vi "OldClimbExecute.vi"(8 "error in (no error)":errorcluster) -> (0 "error out":errorcluster)   [LabVIEW 2023]
uses:
  <vilib>/Rock Robotics/WPI/ThirdParty/JAS_Junk/TrajLib/Trajectory_Library.lvlib
  OldClimbNetworkingGlobal.vi
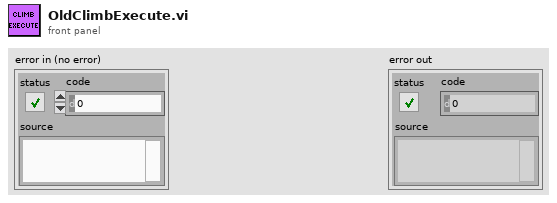
[diagram p1: front panel]
types:
  T1 = typedef "WPI_MotorControlDeviceRef.ctl" = cluster{"DeviceStatus":errorcluster, "Type":T2, "PWM":cluster{"PWM Channel":T3, "DeadBand":T4}, "CAN":cluster{"Device Number":u8, "SetOutput VI Ref":variant, "GetOutput VI Ref":variant, "Enable VI Ref":variant, "Disable VI Ref":variant, "Data":variant}, "Invert":bool, "DIO PWM":cluster{"PWM \"Enable\" Channel":T3, "DIOChannel":T5, "PWM Rate":dbl}}
  T2 = typedef "WPI_MotorControlType.ctl" = enum16{"PWM", "CAN", "DIO PWM"}
  T3 = typedef "FPGA_DIOPWMChannel.ctl" = enum8{"PWM 0", "PWM 1", "PWM 2", "PWM 3", "PWM 4", "PWM 5", "PWM 6", "PWM 7", "PWM 8", "PWM 9", "PWM MXP 0", "PWM MXP 1", "PWM MXP 2", "PWM MXP 3", "PWM MXP 4", "PWM MXP 5", "PWM MXP 6", "PWM MXP 7", "PWM MXP 8", "PWM MXP 9", "Invalid"}
  T4 = typedef "WPI_PWMDeadband.ctl" = cluster{"Name":string, "maxPositivePwm":i32, "minPositivePwm":i32, "centerPwm":i32, "maxNegativePwm":i32, "minNegativePwm":i32, "angularRange":u16}
  T5 = typedef "FPGA_DIOChannel.ctl" = enum8{"DIO 0", "DIO 1", "DIO 2", "DIO 3", "DIO 4", "DIO 5", "DIO 6", "DIO 7", "DIO 8", "DIO 9", "DIO MXP 0", "DIO MXP 1", "DIO MXP 2", "DIO MXP 3", "DIO MXP 4", "DIO MXP 5", "DIO MXP 6", "DIO MXP 7", "DIO MXP 8", "DIO MXP 9", "DIO MXP 10", "DIO MXP 11", "DIO MXP 12", "DIO MXP 13", "DIO MXP 14", "DIO MXP 15", "SPI Port CS1", "SPI Port CS2", "SPI Port CS3", "SPI Port MISO", "SPI Port MOSI", "Invalid"}
  T6 = typedef "Trajectory_Library.lvlib/PosCtrl_Tuning_Type.ctl" = cluster{"Slope":dbl, "Offset":dbl, "Error Deadband":dbl, "At Reference Count":i32, "Negate Output":bool, "Max Allowd Position":dbl, "Min Allowd Position":dbl}
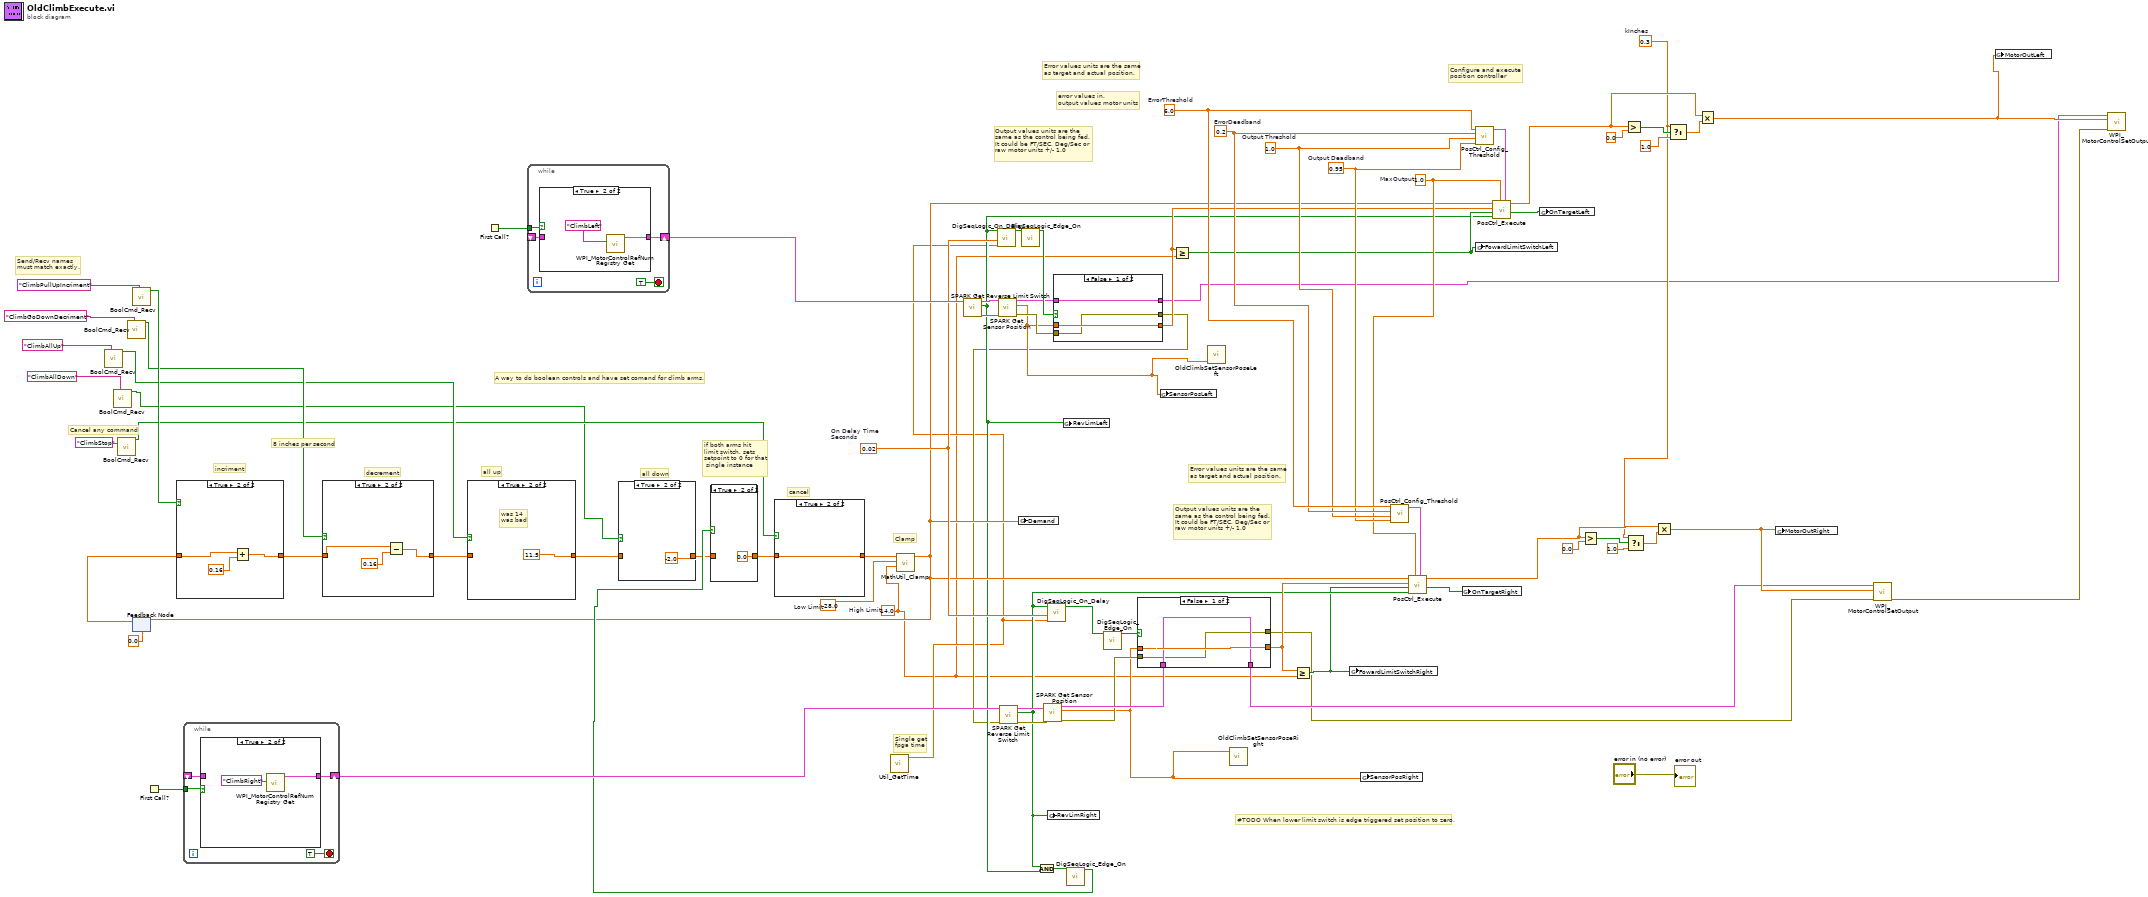
[diagram p0: block diagram]
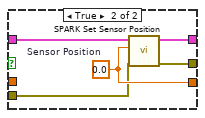
[diagram p5: hidden frame]
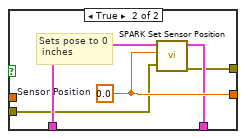
[diagram p6: hidden frame]
diagram:
  w1 = 14.0  # High Limit
  w30 = 0.3  # kInches
  w46 = 0.02  # On Delay Time Seconds
  w62 = -28.0  # Low Limit
  w49 = 1.0  # MaxOutput
  w53 = 6.0  # ErrorThreshold
  w52 = 0.2  # ErrorDeadband
  w51 = 1.0  # Output Threshold
  w50 = 0.95  # Output Deadband
  # "Single get\nfpga time"
  # "if both arms hit \nlimit switch, sets \nsetpoint to 0 for that\n single instance"
  # "#TODO When lower limit switch is edge triggered set position to zero."
  # "cancel"
  # "Clamp"
  # "8 inches per second"
  # "all down"
  # "all up"
  # "decrement"
  # "incriment"
  # "Cancel any command"
  # "Send/Recv names\nmust match exactly."
  # "A way to do boolean controls and have set comand for climb arms."
  # "error values in.\noutput values motor units"
  # "Output values units are the\nsame as the control being fed.  \nIt could be FT/SEC, Deg/Sec or\nraw motor units +/- 1.0"
  # "Error values units are the same \nas target and actual position."
  # "Output values units are the\nsame as the control being fed.  \nIt could be FT/SEC, Deg/Sec or\nraw motor units +/- 1.0"
  # "Error values units are the same \nas target and actual position."
  # "Configure and execute \nposition controller"
  n1 = call <vilib>:"BoolCmd_Recv.vi"("Command Name"="ClimbAllUp") -> ("New Request"=w58:bool)  [unwired: 9 in, 1 out]
  n2 = call <vilib>:"BoolCmd_Recv.vi"("Command Name"="ClimbAllDown") -> ("New Request"=w27:bool)  [unwired: 9 in, 1 out]
  n3 = call <vilib>:"BoolCmd_Recv.vi"("Command Name"="ClimbStop") -> ("New Request"=w57:bool)  [unwired: 9 in, 1 out]
  n4 = call <vilib>:"BoolCmd_Recv.vi"("Command Name"="ClimbGoDownDecriment") -> ("New Request"=w59:bool)  [unwired: 9 in, 1 out]
  n5 = call <vilib>:"BoolCmd_Recv.vi"("Command Name"="ClimbPullUpIncriment") -> ("New Request"=w60:bool)  [unwired: 9 in, 1 out]
  n6 = feedback #1(0.0 ("false")) -> (w66:dbl)
  n7 = First Call?() -> (First Call?: T/F=w24:bool)
  n8 = case shown="True" w60 {
    tunnel: w66 -> [w78 w81]
    tunnel: [w78 w79] -> w65
    frame False {
    }
    frame True {
      n9 = Add(x=w81, y=0.16) -> (x+y=w79:dbl)
    }
  }
  n10 = while {
    tunnel: w24 -> [w84]
    shift-right: [w85] -> w75
    shift-left: _ -> [w83]
    stop <- TRUE stop-if-true
    n11 = case shown="True" w84 {
      tunnel: [w86 w88] -> w85
      tunnel: w83 -> [w86 _]
      frame False {
      }
      frame True {
        n12 = call <vilib>:"WPI_MotorControlRefNum Registry Get.vi"("refnum name"="ClimbRight") -> ("MotorControlDevRef"=w88:T1)  [unwired: 9 in, 1 out]
      }
    }
  }
  n13 = case shown="True" w59 {
    tunnel: w65 -> [w89 w91]
    tunnel: [w89 w90] -> w64
    frame False {
    }
    frame True {
      n14 = Subtract(x=w91, y=0.16) -> (x-y=w90:dbl)
    }
  }
  n15 = case shown="True" w58 {
    tunnel: w64 -> [w93 _]
    tunnel: [w93 11.5 ("y")] -> w63
    frame False {
    }
    frame True {
      # "was 14\nwas bad"
    }
  }
  n16 = First Call?() -> (First Call?: T/F=w23:bool)
  n17 = while {
    tunnel: w23 -> [w97]
    shift-right: [w98] -> w76
    shift-left: _ -> [w96]
    stop <- TRUE stop-if-true
    n18 = case shown="True" w97 {
      tunnel: [w99 w101] -> w98
      tunnel: w96 -> [w99 _]
      frame False {
      }
      frame True {
        n19 = call <vilib>:"WPI_MotorControlRefNum Registry Get.vi"("refnum name"="ClimbLeft") -> ("MotorControlDevRef"=w101:T1)  [unwired: 9 in, 1 out]
      }
    }
  }
  n20 = case shown="True" w27 {
    tunnel: w63 -> [w102 _]
    tunnel: [w102 -2.0 ("y")] -> w26
    frame False {
    }
    frame True {
    }
  }
  n21 = call <vilib>:"Util_GetTime.vi"() -> ("FPGA_Time_Seconds"=w2:dbl)  [unwired: 9 in, 2 out]
  n22 = call <vilib>:"SPARK Get Reverse Limit Switch.vi"("MotorControlDevRef in"=w76) -> ("error out"=w21:errorcluster, "Hard Limit Rev"=w8:bool, "MotorControlDevRef out"=w43:T1)  [unwired: 7 in, 1 out]
  n23 = call <vilib>:"DigSeqLogic_On_Delay.vi"("Time"=w2, "Delay"=w46, "Input"=w8) -> ("Output"=w45:bool)  [unwired: 7 in, 1 out]
  n24 = call <vilib>:"SPARK Get Sensor Position.vi"("error in (no error)"=w21, "MotorControlDevRef in"=w43) -> ("error out"=w20:errorcluster, "Sensor Position"=w7:dbl, "MotorControlDevRef out"=w42:T1)  [unwired: 6 in, 1 out]
  n25 = call <vilib>:"DigSeqLogic_Edge_On.vi"("Input"=w45) -> ("On Edge"=w44:bool)  [unwired: 10 in]
  n26 = case shown="False" w44 {
    tunnel: w42 -> [w106 w111]
    tunnel: [w106 w110] -> w4
    tunnel: w7 -> [w105 _]
    tunnel: [w105 w109] -> w41
    tunnel: w20 -> [w104 w108]
    tunnel: [w104 w107] -> w3
    frame False {
    }
    frame True {
      w109 = 0.0  # Sensor Position
      n27 = call <vilib>:"SPARK Set Sensor Position.vi"("error in"=w108, "Position"=w109, "MotorControlDeviceRef"=w111) -> ("error out"=w107:errorcluster, "MotorControlDeviceRef"=w110:T1)  [unwired: 7 in]
    }
  }
  n28 = call <vilib>:"SPARK Get Reverse Limit Switch.vi"("error in (no error)"=w3, "MotorControlDevRef in"=w75) -> ("error out"=w19:errorcluster, "Hard Limit Rev"=w17:bool, "MotorControlDevRef out"=w74:T1)  [unwired: 6 in, 1 out]
  n29 = And(x=w17, y=w8) -> (x .and. y?=w29:bool)
  n30 = call <vilib>:"SPARK Get Sensor Position.vi"("error in (no error)"=w19, "MotorControlDevRef in"=w74) -> ("error out"=w18:errorcluster, "Sensor Position"=w16:dbl, "MotorControlDevRef out"=w47:T1)  [unwired: 6 in, 1 out]
  n31 = call <vilib>:"DigSeqLogic_On_Delay.vi"("Time"=w2, "Delay"=w46, "Input"=w17) -> ("Output"=w55:bool)  [unwired: 7 in, 1 out]
  n32 = global write "OldClimbNetworkingGlobal.vi" "RevLimRight"(w17) -> ()
  n33 = global write "OldClimbNetworkingGlobal.vi" "RevLimLeft"(w8) -> ()
  n34 = call <vilib>:"DigSeqLogic_Edge_On.vi"("Input"=w29) -> ("On Edge"=w28:bool)  [unwired: 10 in]
  n35 = case shown="True" w28 {
    tunnel: w26 -> [w112 _]
    tunnel: [w112 0.0 ("y")] -> w25
    frame False {
    }
    frame True {
    }
  }
  n36 = case shown="True" w57 {
    tunnel: w25 -> [w114 w115]
    tunnel: [w114 w115] -> w61
    frame False {
    }
    frame True {
    }
  }
  n37 = call <vilib>:"MathUtil_Clamp.vi"("High Limit"=w1, "Low Limit"=w62, "Value"=w61) -> ("Result"=w9:dbl)  [unwired: 8 in]
  n38 = feedback-in #1(w9) -> ()
  n39 = global write "OldClimbNetworkingGlobal.vi" "Demand"(w9) -> ()
  n40 = call <vilib>:"DigSeqLogic_Edge_On.vi"("Input"=w55) -> ("On Edge"=w48:bool)  [unwired: 10 in]
  n41 = case shown="False" w48 {
    tunnel: w16 -> [w118 _]
    tunnel: [w118 w123] -> w54
    tunnel: w47 -> [w117 w122]
    tunnel: [w117 w121] -> w6
    tunnel: w18 -> [w116 w120]
    tunnel: [w116 w119] -> w5
    frame False {
    }
    frame True {
      w123 = 0.0  # Sensor Position
      # "Sets pose to 0\n inches"
      n42 = call <vilib>:"SPARK Set Sensor Position.vi"("error in"=w120, "Position"=w123, "MotorControlDeviceRef"=w122) -> ("error out"=w119:errorcluster, "MotorControlDeviceRef"=w121:T1)  [unwired: 7 in]
    }
  }
  n43 = global write "OldClimbNetworkingGlobal.vi" "SensorPosLeft"(w7) -> ()
  n44 = Greater Or Equal?(x=w41, y=w1) -> (x >= y?=w10:bool)
  n45 = call "OldClimbSetSensorPoseLeft.vi"("ClimbSetSensorPoseLeft"=w7) -> ()  [unwired: 11 in]
  n46 = call "OldClimbSetSensorPoseRight.vi"("ClimbSetSensorPoseRight"=w16) -> ()  [unwired: 11 in]
  n47 = Greater Or Equal?(x=w54, y=w1) -> (x >= y?=w15:bool)
  n48 = global write "OldClimbNetworkingGlobal.vi" "FowardLimitSwitchRight"(w15) -> ()
  n49 = global write "OldClimbNetworkingGlobal.vi" "SensorPosRight"(w16) -> ()
  n50 = call <vilib>:"PosCtrl_Config_Threshold.vi"("Output Deadband"=w50, "Output Threshold"=w51, "ErrorDeadband"=w52, "ErrorThreshold"=w53) -> ("PosCtrl_Config_Params"=w73:T6)  [unwired: 7 in]
  n51 = call <vilib>:"PosCtrl_Execute.vi"("PosCtrl_Config_Params"=w73, "MaxOutput"=w49, "Rev Limit Switch"=w17, "Fwd Limit Switch"=w15, "CurrentPosition"=w54, "TargetPosition"=w9) -> ("OnTarget"=w14:bool, "Output"=w31:dbl)  [unwired: 3 in, 1 out]
  n52 = global write "OldClimbNetworkingGlobal.vi" "OnTargetRight"(w14) -> ()
  n53 = call <vilib>:"PosCtrl_Config_Threshold.vi"("Output Deadband"=w50, "Output Threshold"=w51, "ErrorDeadband"=w52, "ErrorThreshold"=w53) -> ("PosCtrl_Config_Params"=w77:T6)  [unwired: 7 in]
  n54 = global write "OldClimbNetworkingGlobal.vi" "FowardLimitSwitchLeft"(w10) -> ()
  n55 = call <vilib>:"PosCtrl_Execute.vi"("PosCtrl_Config_Params"=w77, "MaxOutput"=w49, "Rev Limit Switch"=w8, "Fwd Limit Switch"=w10, "CurrentPosition"=w41, "TargetPosition"=w9) -> ("OnTarget"=w11:bool, "Output"=w36:dbl)  [unwired: 3 in, 1 out]
  n56 = global write "OldClimbNetworkingGlobal.vi" "OnTargetLeft"(w11) -> ()
  n57 = Greater?(x=w31, y=0.0) -> (0:w34:bool)
  n58 = Greater?(x=w36, y=0.0) -> (0:w39:bool)
  n59 = Select(t=w30, s=w34, f=1.0) -> (s? t:f=w32:dbl)
  n60 = Multiply(x=w31, y=w32) -> (x*y=w13:dbl)
  n61 = Select(t=w30, s=w39, f=1.0) -> (s? t:f=w37:dbl)
  n62 = Multiply(x=w36, y=w37) -> (x*y=w12:dbl)
  n63 = global write "OldClimbNetworkingGlobal.vi" "MotorOutRight"(w13) -> ()
  n64 = call <vilib>:"WPI_MotorControlSetOutput.vi"("error in (no error)"=w5, "Output"=w13, "MotorControlDevRef"=w6) -> ("error out"=w22:errorcluster)  [unwired: 6 in, 2 out]
  n65 = global write "OldClimbNetworkingGlobal.vi" "MotorOutLeft"(w12) -> ()
  n66 = call <vilib>:"WPI_MotorControlSetOutput.vi"("error in (no error)"=w22, "Output"=w12, "MotorControlDevRef"=w4) -> ()  [unwired: 6 in, 3 out]
  "error out" <- "error in (no error)"
